vi "App - analyze RUS V6.vi"() -> ()   [LabVIEW 2021] (continued)
s since 1904-01-01), "Magn Field(T)"=0.0}, {"temperature"=194.69, "lorentzian"={"A (VHz)"=0.0004733372705930792, "ω (Hz)"=665.3791825777425, "Γ (Hz)"=0.12173985621325327, "φ (rad)"=4.657648056590453, "Q"=5465.582129587777, "Norm  Ampl"=0.057880367663565566, "z∞ (V)"=0.5027308717495316-0.030013195107849496i, "4corners"={"z (-pi/2)"=0.0019868048921505323-0.4787308717495316i, "z(inf)"=0.5027308717495316-0.030013195107849496i, "z (pi/2)"=0.05401319510784952+0.4707308717495316i, "z center"=0.028000000000000025-0.0040000000000000036i, "z(0)"=-0.4467308717495316+0.02201319510784949i, "radius"=0.475443042763052}}, "timestamp(min)"=165.23333333432674, "timestamp"=timestamp(3493737735 s since 1904-01-01), "Magn Field(T)"=0.0}, {"temperature"=194.386, "lorentzian"={"A (VHz)"=0.0004690561839457078, "ω (Hz)"=665.3983648536116, "Γ (Hz)"=0.11851104649009389, "φ (rad)"=4.642692437489219, "Q"=5614.652680577173, "Norm  Ampl"=0.056416534703815316, "z∞ (V)"=0.5028887730013848-0.03715180261792456i, "4corners"={"z (-pi/2)"=-0.005151802617924535-0.47888877300138477i, "z(inf)"=0.5028887730013848-0.03715180261792456i, "z (pi/2)"=0.061151802617924585+0.47088877300138476i, "z center"=0.028000000000000025-0.0040000000000000036i, "z(0)"=-0.44688877300138474+0.029151802617924556i, "radius"=0.4760445239046224}}, "timestamp(min)"=166.5666666701436, "timestamp"=timestamp(3493737815 s since 1904-01-01), "Magn Field(T)"=0.0}, {"temperature"=194.091, "lorentzian"={"A (VHz)"=0.00046636153779072714, "ω (Hz)"=665.4185749812924, "Γ (Hz)"=0.11558837012740944, "φ (rad)"=4.620191942670646, "Q"=5756.795205675297, "Norm  Ampl"=0.05515510846662431, "z∞ (V)"=0.49514172142166396-0.04793120585716959i, "4corners"={"z (-pi/2)"=-0.02393120585716957-0.47914172142166395i, "z(inf)"=0.49514172142166396-0.04793120585716959i, "z (pi/2)"=0.0639312058571696+0.47114172142166394i, "z center"=0.020000000000000018-0.0040000000000000036i, "z(0)"=-0.4551417214216639+0.03993120585716958i, "radius"=0.477168320704138}}, "timestamp(min)"=167.88333333283663, "timestamp"=timestamp(3493737894 s since 1904-01-01), "Magn Field(T)"=0.0}, {"temperature"=193.788, "lorentzian"={"A (VHz)"=0.0004694043527923262, "ω (Hz)"=665.4389184365867, "Γ (Hz)"=0.1152399295277775, "φ (rad)"=4.620963148801353, "Q"=5774.378040349192, "Norm  Ampl"=0.05460317404756961, "z∞ (V)"=0.49184277083009437-0.05525921493493594i, "4corners"={"z (-pi/2)"=-0.023259214934935914-0.48384277083009436i, "z(inf)"=0.49184277083009437-0.05525921493493594i, "z (pi/2)"=0.06325921493493594+0.45984277083009434i, "z center"=0.020000000000000018-0.01200000000000001i, "z(0)"=-0.45184277083009433+0.03125921493493592i, "radius"=0.47382165427659373}}, "timestamp(min)"=169.20000000298023, "timestamp"=timestamp(3493737973 s since 1904-01-01), "Magn Field(T)"=0.0}, {"temperature"=193.485, "lorentzian"={"A (VHz)"=0.00046793595663972663, "ω (Hz)"=665.4576110068883, "Γ (Hz)"=0.11547668424833978, "φ (rad)"=4.598129219469584, "Q"=5762.701062456733, "Norm  Ampl"=0.05372182046702751, "z∞ (V)"=0.4901844237391122-0.05704010091712786i, "4corners"={"z (-pi/2)"=-0.025040100917127835-0.4661844237391122i, "z(inf)"=0.4901844237391122-0.05704010091712786i, "z (pi/2)"=0.08104010091712788+0.45818442373911217i, "z center"=0.028000000000000025-0.0040000000000000036i, "z(0)"=-0.43418442373911215+0.049040100917127856i, "radius"=0.46521789932498764}}, "timestamp(min)"=170.5333333313465, "timestamp"=timestamp(3493738053 s since 1904-01-01), "Magn Field(T)"=0.0}, {"temperature"=193.192, "lorentzian"={"A (VHz)"=0.0004687369070369015, "ω (Hz)"=665.4746111668128, "Γ (Hz)"=0.11096973740128416, "φ (rad)"=4.59592026730211, "Q"=5996.901738717747, "Norm  Ampl"=0.051720142968371616, "z∞ (V)"=0.49091673447535344-0.06616043280292741i, "4corners"={"z (-pi/2)"=-0.02616043280292738-0.47491673447535343i, "z(inf)"=0.49091673447535344-0.06616043280292741i, "z (pi/2)"=0.08216043280292742+0.4509167344753534i, "z center"=0.028000000000000025-0.01200000000000001i, "z(0)"=-0.4349167344753534+0.042160432802927396i, "radius"=0.46607430259425936}}, "timestamp(min)"=171.85000000149012, "timestamp"=timestamp(3493738132 s since 1904-01-01), "Magn Field(T)"=0.0}, {"temperature"=192.887, "lorentzian"={"A (VHz)"=0.00047605555056561667, "ω (Hz)"=665.4943966614766, "Γ (Hz)"=0.11194865290221118, "φ (rad)"=4.604033193810438, "Q"=5944.639612973243, "Norm  Ampl"=0.051799398040558914, "z∞ (V)"=0.4879930982279491-0.06203890262826403i, "4corners"={"z (-pi/2)"=-0.022038902628263995-0.4719930982279491i, "z(inf)"=0.4879930982279491-0.06203890262826403i, "z (pi/2)"=0.07803890262826405+0.4479930982279491i, "z center"=0.028000000000000025-0.01200000000000001i, "z(0)"=-0.43199309822794907+0.03803890262826401i, "radius"=0.46270675615727563}}, "timestamp(min)"=173.18333333730698, "timestamp"=timestamp(3493738212 s since 1904-01-01), "Magn Field(T)"=0.0}, {"temperature"=192.594, "lorentzian"={"A (VHz)"=0.0004702108789878097, "ω (Hz)"=665.5130010905406, "Γ (Hz)"=0.10997736867738309, "φ (rad)"=4.5774845869958884, "Q"=6051.363194938885, "Norm  Ampl"=0.05029149690743865, "z∞ (V)"=0.4811346652724541-0.07350341482833078i, "4corners"={"z (-pi/2)"=-0.03350341482833075-0.46513466527245406i, "z(inf)"=0.4811346652724541-0.07350341482833078i, "z (pi/2)"=0.0895034148283308+0.44113466527245404i, "z center"=0.028000000000000025-0.01200000000000001i, "z(0)"=-0.425134665272454+0.04950341482833077i, "radius"=0.4572895088531167}}, "timestamp(min)"=174.5, "timestamp"=timestamp(3493738291 s since 1904-01-01), "Magn Field(T)"=0.0}, {"temperature"=192.288, "lorentzian"={"A (VHz)"=0.0004713592125035609, "ω (Hz)"=665.532316198093, "Γ (Hz)"=0.10978828972623698, "φ (rad)"=4.5635068158593795, "Q"=6061.960869029235, "Norm  Ampl"=0.049822536014935165, "z∞ (V)"=0.47678533676997037-0.07931422899459095i, "4corners"={"z (-pi/2)"=-0.039314228994590916-0.46078533676997036i, "z(inf)"=0.47678533676997037-0.07931422899459095i, "z (pi/2)"=0.09531422899459097+0.43678533676997033i, "z center"=0.028000000000000025-0.01200000000000001i, "z(0)"=-0.4207853367699703+0.05531422899459093i, "radius"=0.45380555739751793}}, "timestamp(min)"=175.8166666701436, "timestamp"=timestamp(3493738370 s since 1904-01-01), "Magn Field(T)"=0.0}, {"temperature"=191.978, "lorentzian"={"A (VHz)"=0.0004778403184541864, "ω (Hz)"=665.5532332931765, "Γ (Hz)"=0.11052784345288488, "φ (rad)"=4.568769136096083, "Q"=6021.5888820529135, "Norm  Ampl"=0.050248078834850406, "z∞ (V)"=0.47793860758755297-0.07706810841072675i, "4corners"={"z (-pi/2)"=-0.03706810841072672-0.46193860758755295i, "z(inf)"=0.47793860758755297-0.07706810841072675i, "z (pi/2)"=0.09306810841072677+0.43793860758755293i, "z center"=0.028000000000000025-0.01200000000000001i, "z(0)"=-0.4219386075875529+0.05306810841072673i, "radius"=0.45461919155483965}}, "timestamp(min)"=177.14999999850988, "timestamp"=timestamp(3493738450 s since 1904-01-01), "Magn Field(T)"=0.0}, {"temperature"=191.681, "lorentzian"={"A (VHz)"=0.0004748373189276945, "ω (Hz)"=665.57156331953, "Γ (Hz)"=0.10923612192313129, "φ (rad)"=4.540652131822902, "Q"=6092.962214347816, "Norm  Ampl"=0.04979499523835774, "z∞ (V)"=0.47714156533718105-0.08190153121076814i, "4corners"={"z (-pi/2)"=-0.04990153121076811-0.45314156533718103i, "z(inf)"=0.47714156533718105-0.08190153121076814i, "z (pi/2)"=0.10590153121076816+0.445141565337181i, "z center"=0.028000000000000025-0.0040000000000000036i, "z(0)"=-0.421141565337181+0.07390153121076813i, "radius"=0.4558473365925434}}, "timestamp(min)"=178.4666666686535, "timestamp"=timestamp(3493738529 s since 1904-01-01), "Magn Field(T)"=0.0}, {"temperature"=191.372, "lorentzian"={"A (VHz)"=0.0004789146193039131, "ω (Hz)"=665.592509513559, "Γ (Hz)"=0.10945268818809382, "φ (rad)"=4.558170526665212, "Q"=6081.097874633669, "Norm  Ampl"=0.04987792297657753, "z∞ (V)"=0.4782947056590417-0.08199957615310491i, "4corners"={"z (-pi/2)"=-0.04199957615310487-0.4622947056590417i, "z(inf)"=0.4782947056590417-0.08199957615310491i, "z (pi/2)"=0.09799957615310492+0.43829470565904166i, "z center"=0.028000000000000025-0.01200000000000001i, "z(0)"=-0.42229470565904165+0.05799957615310489i, "radius"=0.45570304212960583}}, "timestamp(min)"=179.7833333313465, "timestamp"=timestamp(3493738608 s since 1904-01-01), "Magn Field(T)"=0.0}, {"temperature"=191.076, "lorentzian"={"A (VHz)"=0.0004835133622810298, "ω (Hz)"=665.6111561314502, "Γ (Hz)"=0.10913990141816243, "φ (rad)"=4.537491197862966, "Q"=6098.696695548628, "Norm  Ampl"=0.04960117759835196, "z∞ (V)"=0.475540063708298-0.08308176411773265i, "4corners"={"z (-pi/2)"=-0.05108176411773262-0.45154006370829797i, "z(inf)"=0.475540063708298-0.08308176411773265i, "z (pi/2)"=0.10708176411773267+0.44354006370829796i, "z center"=0.028000000000000025-0.0040000000000000036i, "z(0)"=-0.41954006370829794+0.07508176411773264i, "radius"=0.45447335899918284}}, "timestamp(min)"=181.11666666716337, "timestamp"=timestamp(3493738688 s since 1904-01-01), "Magn Field(T)"=0.0}, {"temperature"=190.764, "lorentzian"={"A (VHz)"=0.0004842868501011221, "ω (Hz)"=665.6307876831706, "Γ (Hz)"=0.10814070775046752, "φ (rad)"=4.540583017034438, "Q"=6155.228697218258, "Norm  Ampl"=0.0490010243149022, "z∞ (V)"=0.4744517918520255-0.08946678748136128i, "4corners"={"z (-pi/2)"=-0.04946678748136124-0.4584517918520255i, "z(inf)"=0.4744517918520255-0.08946678748136128i, "z (pi/2)"=0.10546678748136129+0.4344517918520255i, "z center"=0.028000000000000025-0.01200000000000001i, "z(0)"=-0.41845179185202547+0.06546678748136125i, "radius"=0.45312283722029134}}, "timestamp(min)"=182.43333333730698, "timestamp"=timestamp(3493738767 s since 1904-01-01), "Magn Field(T)"=0.0}, {"temperature"=190.453, "lorentzian"={"A (VHz)"=0.00048327521027534057, "ω (Hz)"=665.6495981705524, "Γ (Hz)"=0.10759084438493699, "φ (rad)"=4.513791702941397, "Q"=6186.860991526386, "Norm  Ampl"=0.04861447765885813, "z∞ (V)"=0.47096450993975364-0.09314664631801617i, "4corners"={"z (-pi/2)"=-0.06114664631801614-0.4469645099397536i, "z(inf)"=0.47096450993975364-0.09314664631801617i, "z (pi/2)"=0.11714664631801619+0.4389645099397536i, "z center"=0.028000000000000025-0.0040000000000000036i, "z(0)"=-0.4149645099397536+0.08514664631801616i, "radius"=0.4518458604611926}}, "timestamp(min)"=183.76666666567326, "timestamp"=timestamp(3493738847 s since 1904-01-01), "Magn Field(T)"=0.0}, {"temperature"=190.152, "lorentzian"={"A (VHz)"=0.00047957718786327097, "ω (Hz)"=665.6676827317286, "Γ (Hz)"=0.10502073840326351, "φ (rad)"=4.498887875452793, "Q"=6338.440320002959, "Norm  Ampl"=0.04799160830985852, "z∞ (V)"=0.4665971530227412-0.10082465288267772i, "4corners"={"z (-pi/2)"=-0.0768246528826777-0.45059715302274117i, "z(inf)"=0.4665971530227412-0.10082465288267772i, "z (pi/2)"=0.11682465288267774+0.44259715302274116i, "z center"=0.020000000000000018-0.0040000000000000036i, "z(0)"=-0.42659715302274115+0.09282465288267772i, "radius"=0.45697268024890586}}, "timestamp(min)"=185.08333333581686, "timestamp"=timestamp(3493738926 s since 1904-01-01), "Magn Field(T)"=0.0}, {"temperature"=189.843, "lorentzian"={"A (VHz)"=0.0004830443125643428, "ω (Hz)"=665.6875855513655, "Γ (Hz)"=0.10489848634622057, "φ (rad)"=4.493102336134591, "Q"=6346.017075539526, "Norm  Ampl"=0.04794042267106321, "z∞ (V)"=0.46607304711681385-0.10341652897703693i, "4corners"={"z (-pi/2)"=-0.07941652897703691-0.45007304711681384i, "z(inf)"=0.46607304711681385-0.10341652897703693i, "z (pi/2)"=0.11941652897703695+0.44207304711681383i, "z center"=0.020000000000000018-0.0040000000000000036i, "z(0)"=-0.4260730471168138+0.09541652897703692i, "radius"=0.4570172968257561}}, "timestamp(min)"=186.39999999850988, "timestamp"=timestamp(3493739005 s since 1904-01-01), "Magn Field(T)"=0.0}, {"temperature"=189.545, "lorentzian"={"A (VHz)"=0.00048507486641727196, "ω (Hz)"=665.7073536709393, "Γ (Hz)"=0.10576886336655263, "φ (rad)"=4.485598528155, "Q"=6293.982297643339, "Norm  Ampl"=0.047945199234162496, "z∞ (V)"=0.46969398285832936-0.10592547479419334i, "4corners"={"z (-pi/2)"=-0.07392547479419331-0.44569398285832934i, "z(inf)"=0.46969398285832936-0.10592547479419334i, "z (pi/2)"=0.12992547479419336+0.43769398285832933i, "z center"=0.028000000000000025-0.0040000000000000036i, "z(0)"=-0.4136939828583293+0.09792547479419333i, "radius"=0.4533016400866821}}, "timestamp(min)"=187.73333333432674, "timestamp"=timestamp(3493739085 s since 1904-01-01), "Magn Field(T)"=0.0}, {"temperature"=189.231, "lorentzian"={"A (VHz)"=0.0004854564130087599, "ω (Hz)"=665.7270146903713, "Γ (Hz)"=0.10382219921917683, "φ (rad)"=4.476550298813977, "Q"=6412.18371116344, "Norm  Ampl"=0.04721276914158681, "z∞ (V)"=0.4621584162157943-0.11025537194868097i, "4corners"={"z (-pi/2)"=-0.08625537194868095-0.4461584162157943i, "z(inf)"=0.4621584162157943-0.11025537194868097i, "z (pi/2)"=0.12625537194868097+0.43815841621579427i, "z center"=0.020000000000000018-0.0040000000000000036i, "z(0)"=-0.42215841621579425+0.10225537194868096i, "radius"=0.4547463788733365}}, "timestamp(min)"=189.05000000447035, "timestamp"=timestamp(3493739164 s since 1904-01-01), "Magn Field(T)"=0.0}, {"temperature"=188.914, "lorentzian"={"A (VHz)"=0.000489371270755943, "ω (Hz)"=665.7475776559688, "Γ (Hz)"=0.1035930905389963, "φ (rad)"=4.475172752608208, "Q"=6426.563530367468, "Norm  Ampl"=0.04720162919471164, "z∞ (V)"=0.46288466317147337-0.11107543746185901i, "4corners"={"z (-pi/2)"=-0.08707543746185899-0.44688466317147335i, "z(inf)"=0.46288466317147337-0.11107543746185901i, "z (pi/2)"=0.127075437461859+0.43888466317147334i, "z center"=0.020000000000000018-0.0040000000000000036i, "z(0)"=-0.42288466317147333+0.103075437461859i, "radius"=0.4556445700106146}}, "timestamp(min)"=190.36666666716337, "timestamp"=timestamp(3493739243 s since 1904-01-01), "Magn Field(T)"=0.0}, {"temperature"=188.611, "lorentzian"={"A (VHz)"=0.0004902875733096544, "ω (Hz)"=665.7667570785509, "Γ (Hz)"=0.10246228327177816, "φ (rad)"=4.467488972117573, "Q"=6497.676372413294, "Norm  Ampl"=0.04676865251641132, "z∞ (V)"=0.4628278199416572-0.11466994824295416i, "4corners"={"z (-pi/2)"=-0.09066994824295414-0.4468278199416572i, "z(inf)"=0.4628278199416572-0.11466994824295416i, "z (pi/2)"=0.1306699482429542+0.4388278199416572i, "z center"=0.020000000000000018-0.0040000000000000036i, "z(0)"=-0.4228278199416572+0.10666994824295416i, "radius"=0.45644749485387576}}, "timestamp(min)"=191.70000000298023, "timestamp"=timestamp(3493739323 s since 1904-01-01), "Magn Field(T)"=0.0}, {"temperature"=188.296, "lorentzian"={"A (VHz)"=0.0004887122113930864, "ω (Hz)"=665.7853656920117, "Γ (Hz)"=0.10183598242859536, "φ (rad)"=4.458316232058599, "Q"=6537.820422745393, "Norm  Ampl"=0.04644499941809874, "z∞ (V)"=0.46143498263273536-0.11863393354649247i, "4corners"={"z (-pi/2)"=-0.09463393354649245-0.44543498263273534i, "z(inf)"=0.46143498263273536-0.11863393354649247i, "z (pi/2)"=0.1346339335464925+0.43743498263273534i, "z center"=0.020000000000000018-0.0040000000000000036i, "z(0)"=-0.4214349826327353+0.11063393354649247i, "radius"=0.4560765096037122}}, "timestamp(min)"=193.01666666567326, "timestamp"=timestamp(3493739402 s since 1904-01-01), "Magn Field(T)"=0.0}, {"temperature"=187.992, "lorentzian"={"A (VHz)"=0.000490306698949924, "ω (Hz)"=665.8055568664535, "Γ (Hz)"=0.10204345027139108, "φ (rad)"=4.450722357742632, "Q"=6524.726036758861, "Norm  Ampl"=0.04637710024837498, "z∞ (V)"=0.45901330248316746-0.12157079169587885i, "4corners"={"z (-pi/2)"=-0.09757079169587883-0.44301330248316745i, "z(inf)"=0.45901330248316746-0.12157079169587885i, "z (pi/2)"=0.13757079169587888+0.43501330248316744i, "z center"=0.020000000000000018-0.0040000000000000036i, "z(0)"=-0.4190133024831674+0.11357079169587884i, "radius"=0.4544838509971204}}, "timestamp(min)"=194.35000000149012, "timestamp"=timestamp(3493739482 s since 1904-01-01), "Magn Field(T)"=0.0}, {"temperature"=187.678, "lorentzian"={"A (VHz)"=0.0004933457502481796, "ω (Hz)"=665.8247976415821, "Γ (Hz)"=0.10198962447032296, "φ (rad)"=4.454035586821792, "Q"=6528.358164857489, "Norm  Ampl"=0.04638824792823833, "z∞ (V)"=0.45973800260816855-0.12020480376972283i, "4corners"={"z (-pi/2)"=-0.0962048037697228-0.44373800260816854i, "z(inf)"=0.45973800260816855-0.12020480376972283i, "z (pi/2)"=0.13620480376972283+0.43573800260816853i, "z center"=0.020000000000000018-0.0040000000000000036i, "z(0)"=-0.4197380026081685+0.11220480376972282i, "radius"=0.45483301040819524}}, "timestamp(min)"=195.66666666418314, "timestamp"=timestamp(3493739561 s since 1904-01-01), "Magn Field(T)"=0.0}, {"temperature"=187.365, "lorentzian"={"A (VHz)"=0.0004953119166828639, "ω (Hz)"=665.8450275889691, "Γ (Hz)"=0.10105190378033956, "φ (rad)"=4.4429981058650405, "Q"=6589.138874972036, "Norm  Ampl"=0.04601859160723483, "z∞ (V)"=0.4589709265204048-0.12520095480567314i, "4corners"={"z (-pi/2)"=-0.10120095480567312-0.44297092652040476i, "z(inf)"=0.4589709265204048-0.12520095480567314i, "z (pi/2)"=0.14120095480567316+0.43497092652040475i, "z center"=0.020000000000000018-0.0040000000000000036i, "z(0)"=-0.41897092652040474+0.11720095480567314i, "radius"=0.4553955926180988}}, "timestamp(min)"=196.98333333432674, "timestamp"=timestamp(3493739640 s since 1904-01-01), "Magn Field(T)"=0.0}, {"temperature"=187.059, "lorentzian"={"A (VHz)"=0.0004971004064286509, "ω (Hz)"=665.8652215366186, "Γ (Hz)"=0.10124311654960735, "φ (rad)"=4.44477946117701, "Q"=6576.893760578343, "Norm  Ampl"=0.045756849533585525, "z∞ (V)"=0.4558634017071746-0.12350775278993242i, "4corners"={"z (-pi/2)"=-0.0995077527899324-0.4398634017071746i, "z(inf)"=0.4558634017071746-0.12350775278993242i, "z (pi/2)"=0.13950775278993244+0.4318634017071746i, "z center"=0.020000000000000018-0.0040000000000000036i, "z(0)"=-0.41586340170717456+0.11550775278993242i, "radius"=0.4519502272647392}}, "timestamp(min)"=198.3166666701436, "timestamp"=timestamp(3493739720 s since 1904-01-01), "Magn Field(T)"=0.0}, {"temperature"=186.735, "lorentzian"={"A (VHz)"=0.0004972570590289756, "ω (Hz)"=665.8855803249663, "Γ (Hz)"=0.1006065069019078, "φ (rad)"=4.429091539266533, "Q"=6618.712852978888, "Norm  Ampl"=0.045593672054500184, "z∞ (V)"=0.455123549159136-0.13067657260833146i, "4corners"={"z (-pi/2)"=-0.10667657260833144-0.439123549159136i, "z(inf)"=0.455123549159136-0.13067657260833146i, "z (pi/2)"=0.14667657260833147+0.431123549159136i, "z center"=0.020000000000000018-0.0040000000000000036i, "z(0)"=-0.41512354915913596+0.12267657260833145i, "radius"=0.45318810341913973}}, "timestamp(min)"=199.63333333283663, "timestamp"=timestamp(3493739799 s since 1904-01-01), "Magn Field(T)"=0.0}, {"temperature"=186.417, "lorentzian"={"A (VHz)"=0.0005019454828646748, "ω (Hz)"=665.9069182376624, "Γ (Hz)"=0.10072773069953611, "φ (rad)"=4.429879213030441, "Q"=6610.959202724589, "Norm  Ampl"=0.04551935260615651, "z∞ (V)"=0.4539908347721079-0.1299760766146092i, "4corners"={"z (-pi/2)"=-0.10597607661460917-0.4379908347721079i, "z(inf)"=0.4539908347721079-0.1299760766146092i, "z (pi/2)"=0.1459760766146092+0.42999083477210787i, "z center"=0.020000000000000018-0.0040000000000000036i, "z(0)"=-0.41399083477210785+0.12197607661460919i, "radius"=0.451904875549491}}, "timestamp(min)"=200.95000000298023, "timestamp"=timestamp(3493739878 s since 1904-01-01), "Magn Field(T)"=0.0}, {"temperature"=186.086, "lorentzian"={"A (VHz)"=0.0005031496956658738, "ω (Hz)"=665.9269377443005, "Γ (Hz)"=0.10071825546470319, "φ (rad)"=4.417121585751774, "Q"=6611.779906947209, "Norm  Ampl"=0.04536722950947459, "z∞ (V)"=0.45094405956642014-0.13507522462523452i, "4corners"={"z (-pi/2)"=-0.1110752246252345-0.4349440595664201i, "z(inf)"=0.45094405956642014-0.13507522462523452i, "z (pi/2)"=0.15107522462523454+0.4269440595664201i, "z center"=0.020000000000000018-0.0040000000000000036i, "z(0)"=-0.4109440595664201+0.12707522462523452i, "radius"=0.4504370066792269}}, "timestamp(min)"=202.2833333313465, "timestamp"=timestamp(3493739958 s since 1904-01-01), "Magn Field(T)"=0.0}, {"temperature"=185.758, "lorentzian"={"A (VHz)"=0.0005026440005685532, "ω (Hz)"=665.9465552746622, "Γ (Hz)"=0.09998730289056303, "φ (rad)"=4.418941189120801, "Q"=6660.311219751036, "Norm  Ampl"=0.04509680832517295, "z∞ (V)"=0.4517450443366491-0.1344610417899304i, "4corners"={"z (-pi/2)"=-0.11046104178993038-0.43574504433664907i, "z(inf)"=0.4517450443366491-0.1344610417899304i, "z (pi/2)"=0.15046104178993042+0.42774504433664906i, "z center"=0.020000000000000018-0.0040000000000000036i, "z(0)"=-0.41174504433664905+0.1264610417899304i, "radius"=0.45102535043406267}}, "timestamp(min)"=203.60000000149012, "timestamp"=timestamp(3493740037 s since 1904-01-01), "Magn Field(T)"=0.0}, {"temperature"=185.416, "lorentzian"={"A (VHz)"=0.0005040996879191407, "ω (Hz)"=665.9681031960093, "Γ (Hz)"=0.09919861575064098, "φ (rad)"=4.41637602527476, "Q"=6713.481817831778, "Norm  Ampl"=0.04474333988174422, "z∞ (V)"=0.4514306602736386-0.13557472298986503i, "4corners"={"z (-pi/2)"=-0.11157472298986501-0.4354306602736386i, "z(inf)"=0.4514306602736386-0.13557472298986503i, "z (pi/2)"=0.15157472298986505+0.4274306602736386i, "z center"=0.020000000000000018-0.0040000000000000036i, "z(0)"=-0.41143066027363856+0.12757472298986502i, "radius"=0.4510480266601412}}, "timestamp(min)"=204.93333333730698, "timestamp"=timestamp(3493740117 s since 1904-01-01), "Magn Field(T)"=0.0}, {"temperature"=185.07, "lorentzian"={"A (VHz)"=0.0005067104672487048, "ω (Hz)"=665.9882719429886, "Γ (Hz)"=0.0995403994380663, "φ (rad)"=4.40693887801457, "Q"=6690.6329058621495, "Norm  Ampl"=0.04476557949293247, "z∞ (V)"=0.4489058197470238-0.13924172969995527i, "4corners"={"z (-pi/2)"=-0.11524172969995525-0.4329058197470238i, "z(inf)"=0.4489058197470238-0.13924172969995527i, "z (pi/2)"=0.15524172969995528+0.4249058197470238i, "z center"=0.020000000000000018-0.0040000000000000036i, "z(0)"=-0.4089058197470238+0.13124172969995526i, "radius"=0.4497227230917982}}, "timestamp(min)"=206.25, "timestamp"=timestamp(3493740196 s since 1904-01-01), "Magn Field(T)"=0.0}, {"temperature"=184.744, "lorentzian"={"A (VHz)"=0.0005112253916703258, "ω (Hz)"=666.0103637387408, "Γ (Hz)"=0.09881436622074807, "φ (rad)"=4.408059992114199, "Q"=6740.015538336757, "Norm  Ampl"=0.04467483988391522, "z∞ (V)"=0.4513335591459692-0.1394757736017544i, "4corners"={"z (-pi/2)"=-0.11547577360175437-0.43533355914596916i, "z(inf)"=0.4513335591459692-0.1394757736017544i, "z (pi/2)"=0.1554757736017544+0.42733355914596916i, "z center"=0.020000000000000018-0.0040000000000000036i, "z(0)"=-0.41133355914596914+0.1314757736017544i, "radius"=0.45210875293287905}}, "timestamp(min)"=207.5666666701436, "timestamp"=timestamp(3493740275 s since 1904-01-01), "Magn Field(T)"=0.0}, {"temperature"=184.426, "lorentzian"={"A (VHz)"=0.000507371909104018, "ω (Hz)"=666.0300130208008, "Γ (Hz)"=0.09810406651763616, "φ (rad)"=4.396204108196729, "Q"=6789.015345261642, "Norm  Ampl"=0.04407972986050783, "z∞ (V)"=0.4470428153414331-0.1437115965133239i, "4corners"={"z (-pi/2)"=-0.11971159651332389-0.43104281534143307i, "z(inf)"=0.4470428153414331-0.1437115965133239i, "z (pi/2)"=0.15971159651332392+0.42304281534143306i, "z center"=0.020000000000000018-0.0040000000000000036i, "z(0)"=-0.40704281534143305+0.1357115965133239i, "radius"=0.4493160316915468}}, "timestamp(min)"=208.89999999850988, "timestamp"=timestamp(3493740355 s since 1904-01-01), "Magn Field(T)"=0.0}, {"temperature"=184.132, "lorentzian"={"A (VHz)"=0.000505511013373246, "ω (Hz)"=666.0483020662261, "Γ (Hz)"=0.09733473734784187, "φ (rad)"=4.383921206579432, "Q"=6842.863300550057, "Norm  Ampl"=0.04345140554070788, "z∞ (V)"=0.44254591035348945-0.1480094656405301i, "4corners"={"z (-pi/2)"=-0.12400946564053009-0.42654591035348943i, "z(inf)"=0.44254591035348945-0.1480094656405301i, "z (pi/2)"=0.16400946564053012+0.4185459103534894i, "z center"=0.020000000000000018-0.0040000000000000036i, "z(0)"=-0.4025459103534894+0.1400094656405301i, "radius"=0.446412110667408}}, "timestamp(min)"=210.2166666686535, "timestamp"=timestamp(3493740434 s since 1904-01-01), "Magn Field(T)"=0.0}, {"temperature"=183.85, "lorentzian"={"A (VHz)"=0.0005107537794322983, "ω (Hz)"=666.067358184188, "Γ (Hz)"=0.09764163972161045, "φ (rad)"=4.378344884681519, "Q"=6821.550314837362, "Norm  Ampl"=0.04352088907430267, "z∞ (V)"=0.4410830036631965-0.15013673950216963i, "4corners"={"z (-pi/2)"=-0.1261367395021696-0.4250830036631965i, "z(inf)"=0.4410830036631965-0.15013673950216963i, "z (pi/2)"=0.16613673950216964+0.4170830036631965i, "z center"=0.020000000000000018-0.0040000000000000036i, "z(0)"=-0.4010830036631965+0.14213673950216962i, "radius"=0.4457205880440621}}, "timestamp(min)"=211.5333333313465, "timestamp"=timestamp(3493740513 s since 1904-01-01), "Magn Field(T)"=0.0}, {"temperature"=183.537, "lorentzian"={"A (VHz)"=0.0005135418857311315, "ω (Hz)"=666.0861004254415, "Γ (Hz)"=0.09757767007940571, "φ (rad)"=4.370614067546287, "Q"=6826.214439055586, "Norm  Ampl"=0.04336398599881979, "z∞ (V)"=0.43870100097708137-0.15294666005538513i, "4corners"={"z (-pi/2)"=-0.1289466600553851-0.42270100097708135i, "z(inf)"=0.43870100097708137-0.15294666005538513i, "z (pi/2)"=0.16894666005538514+0.41470100097708135i, "z center"=0.020000000000000018-0.0040000000000000036i, "z(0)"=-0.39870100097708133+0.14494666005538512i, "radius"=0.44440481068600546}}, "timestamp(min)"=212.86666666716337, "timestamp"=timestamp(3493740593 s since 1904-01-01), "Magn Field(T)"=0.0}, {"temperature"=183.227, "lorentzian"={"A (VHz)"=0.00051361107923451, "ω (Hz)"=666.1047052834762, "Γ (Hz)"=0.09706117767337244, "φ (rad)"=4.365948479035594, "Q"=6862.7305092570905, "Norm  Ampl"=0.04326187056886954, "z∞ (V)"=0.4392362710126165-0.15534426252176073i, "4corners"={"z (-pi/2)"=-0.1313442625217607-0.42323627101261646i, "z(inf)"=0.4392362710126165-0.15534426252176073i, "z (pi/2)"=0.17134426252176074+0.41523627101261645i, "z center"=0.020000000000000018-0.0040000000000000036i, "z(0)"=-0.39923627101261644+0.14734426252176072i, "radius"=0.44571755263935886}}, "timestamp(min)"=214.18333333730698, "timestamp"=timestamp(3493740672 s since 1904-01-01), "Magn Field(T)"=0.0}, {"temperature"=182.898, "lorentzian"={"A (VHz)"=0.0004955884328845794, "ω (Hz)"=666.12482136998, "Γ (Hz)"=0.0785871229872767, "φ (rad)"=4.3809115704954245, "Q"=8476.259163703271, "Norm  Ampl"=0.04130830816306614, "z∞ (V)"=0.4290227743933384-0.16706353355510292i, "4corners"={"z (-pi/2)"=-0.23906353355510293-0.4930227743933384i, "z(inf)"=0.4290227743933384-0.16706353355510292i, "z (pi/2)"=0.10306353355510292+0.5010227743933384i, "z center"=-0.068+0.0040000000000000036i, "z(0)"=-0.5650227743933385+0.17506353355510293i, "radius"=0.5256371093996401}}, "timestamp(min)"=215.5, "timestamp"=timestamp(3493740751 s since 1904-01-01), "Magn Field(T)"=0.0}, {"temperature"=182.567, "lorentzian"={"A (VHz)"=0.0004957520657761678, "ω (Hz)"=666.140704057652, "Γ (Hz)"=0.07744723171787302, "φ (rad)"=4.342947303070082, "Q"=8601.220331338483, "Norm  Ampl"=0.040979781525970205, "z∞ (V)"=0.4254306607295709-0.1790667065333622i, "4corners"={"z (-pi/2)"=-0.2590667065333622-0.4814306607295709i, "z(inf)"=0.4254306607295709-0.1790667065333622i, "z (pi/2)"=0.12306670653336221+0.5054306607295709i, "z center"=-0.068+0.01200000000000001i, "z(0)"=-0.5614306607295709+0.20306670653336223i, "radius"=0.5291316502473906}}, "timestamp(min)"=216.83333333581686, "timestamp"=timestamp(3493740831 s since 1904-01-01), "Magn Field(T)"=0.0}, {"temperature"=182.25, "lorentzian"={"A (VHz)"=0.0005041586824842459, "ω (Hz)"=666.1610854922133, "Γ (Hz)"=0.07919201632548688, "φ (rad)"=4.345514661958893, "Q"=8411.972777081803, "Norm  Ampl"=0.04150138086075732, "z∞ (V)"=0.4211855739536328-0.18398012408312936i, "4corners"={"z (-pi/2)"=-0.25598012408312937-0.4851855739536328i, "z(inf)"=0.4211855739536328-0.18398012408312936i, "z (pi/2)"=0.11998012408312936+0.4931855739536328i, "z center"=-0.068+0.0040000000000000036i, "z(0)"=-0.5571855739536329+0.19198012408312937i, "radius"=0.5240601614458534}}, "timestamp(min)"=218.14999999850988, "timestamp"=timestamp(3493740910 s since 1904-01-01), "Magn Field(T)"=0.0}, {"temperature"=181.923, "lorentzian"={"A (VHz)"=0.0004993870496341144, "ω (Hz)"=666.1802100253361, "Γ (Hz)"=0.07801021052157167, "φ (rad)"=4.331869513816752, "Q"=8539.65404748038, "Norm  Ampl"=0.04137904366180594, "z∞ (V)"=0.42449035626147175-0.1850036204032826i, "4corners"={"z (-pi/2)"=-0.2650036204032826-0.48049035626147174i, "z(inf)"=0.42449035626147175-0.1850036204032826i, "z (pi/2)"=0.12900362040328262+0.5044903562614718i, "z center"=-0.068+0.01200000000000001i, "z(0)"=-0.5604903562614718+0.20900362040328263i, "radius"=0.5304311241457764}}, "timestamp(min)"=219.48333333432674, "timestamp"=timestamp(3493740990 s since 1904-01-01), "Magn Field(T)"=0.0}, {"temperature"=181.605, "lorentzian"={"A (VHz)"=0.0005167479944593708, "ω (Hz)"=666.2003193033272, "Γ (Hz)"=0.09635905306280869, "φ (rad)"=4.338129044767257, "Q"=6913.7283745315035, "Norm  Ampl"=0.042748236252394184, "z∞ (V)"=0.4329257714649433-0.16618571965142953i, "4corners"={"z (-pi/2)"=-0.1421857196514295-0.4169257714649433i, "z(inf)"=0.4329257714649433-0.16618571965142953i, "z (pi/2)"=0.18218571965142955+0.4089257714649433i, "z center"=0.020000000000000018-0.0040000000000000036i, "z(0)"=-0.3929257714649433+0.15818571965142952i, "radius"=0.4436348728388816}}, "timestamp(min)"=220.80000000447035, "timestamp"=timestamp(3493741069 s since 1904-01-01), "Magn Field(T)"=0.0}, {"temperature"=181.283, "lorentzian"={"A (VHz)"=0.0005026422229183416, "ω (Hz)"=666.2201606193609, "Γ (Hz)"=0.07853309652980567, "φ (rad)"=4.3272218352270935, "Q"=8483.304365395936, "Norm  Ampl"=0.041422115997539526, "z∞ (V)"=0.4208047607766637-0.1861695780664665i, "4corners"={"z (-pi/2)"=-0.2661695780664665-0.47680476077666367i, "z(inf)"=0.4208047607766637-0.1861695780664665i, "z (pi/2)"=0.1301695780664665+0.5008047607766637i, "z center"=-0.068+0.01200000000000001i, "z(0)"=-0.5568047607766637+0.21016957806646652i, "radius"=0.5274478892070503}}, "timestamp(min)"=222.11666666716337, "timestamp"=timestamp(3493741148 s since 1904-01-01), "Magn Field(T)"=0.0}, {"temperature"=180.967, "lorentzian"={"A (VHz)"=0.0005215234623542747, "ω (Hz)"=666.23899502151, "Γ (Hz)"=0.09689739098125703, "φ (rad)"=4.324067544116355, "Q"=6875.716552062598, "Norm  Ampl"=0.04309277988443051, "z∞ (V)"=0.4316142499095974-0.17238895373709437i, "4corners"={"z (-pi/2)"=-0.14838895373709435-0.4156142499095974i, "z(inf)"=0.4316142499095974-0.17238895373709437i, "z (pi/2)"=0.18838895373709438+0.4076142499095974i, "z center"=0.020000000000000018-0.0040000000000000036i, "z(0)"=-0.39161424990959737+0.16438895373709436i, "radius"=0.4447259048777278}}, "timestamp(min)"=223.45000000298023, "timestamp"=timestamp(3493741228 s since 1904-01-01), "Magn Field(T)"=0.0}, {"temperature"=180.662, "lorentzian"={"A (VHz)"=0.0005212480476639817, "ω (Hz)"=666.257459442358, "Γ (Hz)"=0.09678513871433185, "φ (rad)"=4.317919649999137, "Q"=6883.881846869733, "Norm  Ampl"=0.04314651939659813, "z∞ (V)"=0.43156002736862603-0.17532793765444946i, "4corners"={"z (-pi/2)"=-0.15132793765444943-0.415560027368626i, "z(inf)"=0.43156002736862603-0.17532793765444946i, "z (pi/2)"=0.19132793765444947+0.407560027368626i, "z center"=0.020000000000000018-0.0040000000000000036i, "z(0)"=-0.391560027368626+0.16732793765444945i, "radius"=0.44579694744198406}}, "timestamp(min)"=224.76666666567326, "timestamp"=timestamp(3493741307 s since 1904-01-01), "Magn Field(T)"=0.0}, {"temperature"=180.335, "lorentzian"={"A (VHz)"=0.0005249035648374328, "ω (Hz)"=666.2778888148354, "Γ (Hz)"=0.09695910604151245, "φ (rad)"=4.320044957943992, "Q"=6871.741252746004, "Norm  Ampl"=0.04310261203432272, "z∞ (V)"=0.4307657006363299-0.173973879869461i, "4corners"={"z (-pi/2)"=-0.14997387986946098-0.4147657006363299i, "z(inf)"=0.4307657006363299-0.173973879869461i, "z (pi/2)"=0.18997387986946102+0.4067657006363299i, "z center"=0.020000000000000018-0.0040000000000000036i, "z(0)"=-0.39076570063632987+0.165973879869461i, "radius"=0.4445442392576165}}, "timestamp(min)"=226.08333333581686, "timestamp"=timestamp(3493741386 s since 1904-01-01), "Magn Field(T)"=0.0}, {"temperature"=180.012, "lorentzian"={"A (VHz)"=0.0005280581772481593, "ω (Hz)"=666.2970981562802, "Γ (Hz)"=0.09685494012184559, "φ (rad)"=4.3088833285164, "Q"=6879.330030229374, "Norm  Ampl"=0.043348671110678284, "z∞ (V)"=0.43161913617069037-0.1797332456610516i, "4corners"={"z (-pi/2)"=-0.15573324566105157-0.41561913617069035i, "z(inf)"=0.43161913617069037-0.1797332456610516i, "z (pi/2)"=0.1957332456610516+0.40761913617069034i, "z center"=0.020000000000000018-0.0040000000000000036i, "z(0)"=-0.39161913617069033+0.17173324566105158i, "radius"=0.4475628301059783}}, "timestamp(min)"=227.41666666418314, "timestamp"=timestamp(3493741466 s since 1904-01-01), "Magn Field(T)"=0.0}, {"temperature"=179.664, "lorentzian"={"A (VHz)"=0.0005290576023142959, "ω (Hz)"=666.3156869001568, "Γ (Hz)"=0.0968776485916216, "φ (rad)"=4.305407122936881, "Q"=6877.909369053191, "Norm  Ampl"=0.043264476719602526, "z∞ (V)"=0.43011133132964025-0.1807775100196454i, "4corners"={"z (-pi/2)"=-0.15677751001964538-0.41411133132964023i, "z(inf)"=0.43011133132964025-0.1807775100196454i, "z (pi/2)"=0.1967775100196454+0.4061113313296402i, "z center"=0.020000000000000018-0.0040000000000000036i, "z(0)"=-0.3901113313296402+0.1727775100196454i, "radius"=0.44658884013566186}}, "timestamp(min)"=228.73333333432674, "timestamp"=timestamp(3493741545 s since 1904-01-01), "Magn Field(T)"=0.0}, {"temperature"=179.311, "lorentzian"={"A (VHz)"=0.0005260404663695264, "ω (Hz)"=666.3357577270784, "Γ (Hz)"=0.09648267448631179, "φ (rad)"=4.290413592229389, "Q"=6906.273704317898, "Norm  Ampl"=0.04319321345949962, "z∞ (V)"=0.42840883917162537-0.18735268780586156i, "4corners"={"z (-pi/2)"=-0.16335268780586154-0.41240883917162535i, "z(inf)"=0.42840883917162537-0.18735268780586156i, "z (pi/2)"=0.20335268780586158+0.40440883917162534i, "z center"=0.020000000000000018-0.0040000000000000036i, "z(0)"=-0.38840883917162533+0.17935268780586155i, "radius"=0.44767844267861306}}, "timestamp(min)"=230.0666666701436, "timestamp"=timestamp(3493741625 s since 1904-01-01), "Magn Field(T)"=0.0}, {"temperature"=178.96, "lorentzian"={"A (VHz)"=0.0005258544343686757, "ω (Hz)"=666.3558831541329, "Γ (Hz)"=0.09658600169222692, "φ (rad)"=4.288747421238792, "Q"=6899.093776316451, "Norm  Ampl"=0.043267147821974376, "z∞ (V)"=0.42836399654767815-0.18815070892141575i, "4corners"={"z (-pi/2)"=-0.16415070892141573-0.41236399654767814i, "z(inf)"=0.42836399654767815-0.18815070892141575i, "z (pi/2)"=0.20415070892141576+0.40436399654767813i, "z center"=0.020000000000000018-0.0040000000000000036i, "z(0)"=-0.3883639965476781+0.18015070892141574i, "radius"=0.4479649955885527}}, "timestamp(min)"=231.38333333283663, "timestamp"=timestamp(3493741704 s since 1904-01-01), "Magn Field(T)"=0.0}, {"temperature"=178.579, "lorentzian"={"A (VHz)"=0.0005230376437687634, "ω (Hz)"=666.3762094650621, "Γ (Hz)"=0.09539125746584712, "φ (rad)"=4.26202904676002, "Q"=6985.715747626499, "Norm  Ampl"=0.0428746982316789, "z∞ (V)"=0.4246459172867293-0.19164592232429825i, "4corners"={"z (-pi/2)"=-0.17564592232429824-0.40064591728672927i, "z(inf)"=0.4246459172867293-0.19164592232429825i, "z (pi/2)"=0.21564592232429827+0.4086459172867293i, "z center"=0.020000000000000018+0.0040000000000000036i, "z(0)"=-0.38464591728672926+0.19964592232429826i, "radius"=0.44946150591451534}}, "timestamp(min)"=232.70000000298023, "timestamp"=timestamp(3493741783 s since 1904-01-01), "Magn Field(T)"=0.0}, {"temperature"=178.21, "lorentzian"={"A (VHz)"=0.0005259446589709141, "ω (Hz)"=666.3976643168794, "Γ (Hz)"=0.0958751148522994, "φ (rad)"=4.273866226248172, "Q"=6950.684391288602, "Norm  Ampl"=0.04311541821371235, "z∞ (V)"=0.427152917559753-0.19494540509248812i, "4corners"={"z (-pi/2)"=-0.1709454050924881-0.411152917559753i, "z(inf)"=0.427152917559753-0.19494540509248812i, "z (pi/2)"=0.21094540509248813+0.40315291755975297i, "z center"=0.020000000000000018-0.0040000000000000036i, "z(0)"=-0.38715291755975295+0.1869454050924881i, "radius"=0.4497039537332904}}, "timestamp(min)"=234.0333333313465, "timestamp"=timestamp(3493741863 s since 1904-01-01), "Magn Field(T)"=0.0}, {"temperature"=177.848, "lorentzian"={"A (VHz)"=0.0005279001236632242, "ω (Hz)"=666.4187151485258, "Γ (Hz)"=0.09636441325121417, "φ (rad)"=4.253053034777806, "Q"=6915.61015798671, "Norm  Ampl"=0.04326563911074433, "z∞ (V)"=0.4224414104926588-0.20305636790907744i, "4corners"={"z (-pi/2)"=-0.17905636790907742-0.4064414104926588i, "z(inf)"=0.4224414104926588-0.20305636790907744i, "z (pi/2)"=0.21905636790907745+0.3984414104926588i, "z center"=0.020000000000000018-0.0040000000000000036i, "z(0)"=-0.3824414104926588+0.19505636790907743i, "radius"=0.4489794276851387}}, "timestamp(min)"=235.35000000149012, "timestamp"=timestamp(3493741942 s since 1904-01-01), "Magn Field(T)"=0.0}, {"temperature"=177.556, "lorentzian"={"A (VHz)"=0.0005262689635044686, "ω (Hz)"=666.4383021086978, "Γ (Hz)"=0.09521086614962272, "φ (rad)"=4.242752376599923, "Q"=6999.603396753036, "Norm  Ampl"=0.04285992485305398, "z∞ (V)"=0.4214205796099437-0.19972448403641094i, "4corners"={"z (-pi/2)"=-0.18372448403641092-0.3974205796099437i, "z(inf)"=0.4214205796099437-0.19972448403641094i, "z (pi/2)"=0.22372448403641096+0.4054205796099437i, "z center"=0.020000000000000018+0.0040000000000000036i, "z(0)"=-0.3814205796099437+0.20772448403641094i, "radius"=0.45015791354844026}}, "timestamp(min)"=236.66666666418314, "timestamp"=timestamp(3493742021 s since 1904-01-01), "Magn Field(T)"=0.0}, {"temperature"=177.306, "lorentzian"={"A (VHz)"=0.0005237589663709974, "ω (Hz)"=666.4551854285005, "Γ (Hz)"=0.09491832663958324, "φ (rad)"=4.229125837747038, "Q"=7021.3541370057455, "Norm  Ampl"=0.04280145372354218, "z∞ (V)"=0.4192903798882296-0.2055338108907991i, "4corners"={"z (-pi/2)"=-0.1895338108907991-0.39529037988822957i, "z(inf)"=0.4192903798882296-0.2055338108907991i, "z (pi/2)"=0.22953381089079913+0.4032903798882296i, "z center"=0.020000000000000018+0.0040000000000000036i, "z(0)"=-0.37929037988822956+0.21353381089079912i, "radius"=0.4509292908846218}}, "timestamp(min)"=238.0, "timestamp"=timestamp(3493742101 s since 1904-01-01), "Magn Field(T)"=0.0}, {"temperature"=177.009, "lorentzian"={"A (VHz)"=0.0005248334524811574, "ω (Hz)"=666.4720190334131, "Γ (Hz)"=0.09480054002810678, "φ (rad)"=4.221662538561555, "Q"=7030.25551158058, "Norm  Ampl"=0.042607464000126286, "z∞ (V)"=0.4164047972828688-0.20780765549778904i, "4corners"={"z (-pi/2)"=-0.19180765549778903-0.39240479728286876i, "z(inf)"=0.4164047972828688-0.20780765549778904i, "z (pi/2)"=0.23180765549778906+0.40040479728286876i, "z center"=0.020000000000000018+0.0040000000000000036i, "z(0)"=-0.37640479728286874+0.21580765549778905i, "radius"=0.4494432625330392}}, "timestamp(min)"=239.3166666701436, "timestamp"=timestamp(3493742180 s since 1904-01-01), "Magn Field(T)"=0.0}, {"temperature"=176.677, "lorentzian"={"A (VHz)"=0.0005261115498054191, "ω (Hz)"=666.4896912216159, "Γ (Hz)"=0.09527454689557305, "φ (rad)"=4.212516438506931, "Q"=6995.464297008212, "Norm  Ampl"=0.04291764550443332, "z∞ (V)"=0.4153458795475509-0.21191301413046024i, "4corners"={"z (-pi/2)"=-0.19591301413046022-0.3913458795475509i, "z(inf)"=0.4153458795475509-0.21191301413046024i, "z (pi/2)"=0.23591301413046026+0.3993458795475509i, "z center"=0.020000000000000018+0.0040000000000000036i, "z(0)"=-0.3753458795475509+0.21991301413046024i, "radius"=0.4504628665563089}}, "timestamp(min)"=240.63333333283663, "timestamp"=timestamp(3493742259 s since 1904-01-01), "Magn Field(T)"=0.0}, {"temperature"=176.315, "lorentzian"={"A (VHz)"=0.0005256117490866303, "ω (Hz)"=666.5084730527226, "Γ (Hz)"=0.09408649571724803, "φ (rad)"=4.207063834838992, "Q"=7083.997208863392, "Norm  Ampl"=0.042629920830408, "z∞ (V)"=0.4164640226070026-0.2153386241198867i, "4corners"={"z (-pi/2)"=-0.19933862411988668-0.3924640226070026i, "z(inf)"=0.4164640226070026-0.2153386241198867i, "z (pi/2)"=0.2393386241198867+0.4004640226070026i, "z center"=0.020000000000000018+0.0040000000000000036i, 
